vi "ReadGroupedDigitalOutputs.vi"(8 "error in (no error)":errorcluster, 11 "TesteractHAL_DigitalOutput_NIDAQmx In":refnum<class "TesteractHAL_DigitalOutput_NIDAQmx.lvclass">) -> (0 "error out":errorcluster, 2 "data":u32, 3 "TesteractHAL_DigitalOutput_NIDAQmx Out":refnum<class "TesteractHAL_DigitalOutput_NIDAQmx.lvclass">)   [LabVIEW 2017, in "TesteractHAL_DigitalOutput_NIDAQmx.lvlib" / "TesteractHAL_DigitalOutput_NIDAQmx.lvclass"]
doc: "Read a single channel."
uses:
  TesteractHAL_DigitalOutput_NIDAQmx.lvclass
  TesteractHAL_DigitalOutput_NIDAQmx.lvclass/TesteractHAL_DigitalOutput_NIDAQmx.ctl
  <vilib>/DAQmx/read.llb/DAQmx Read (Digital U32 1Chan 1Samp).vi
  <vilib>/DAQmx/miscellaneous.llb/DAQmx Fill In Error Info.vi
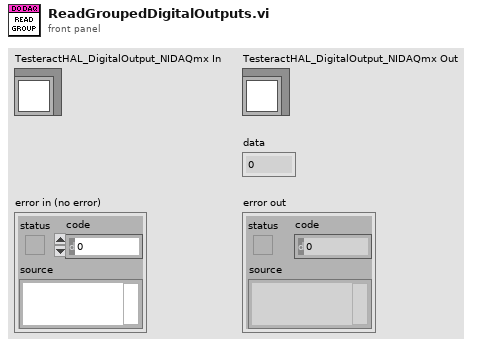
[diagram p1: front panel]
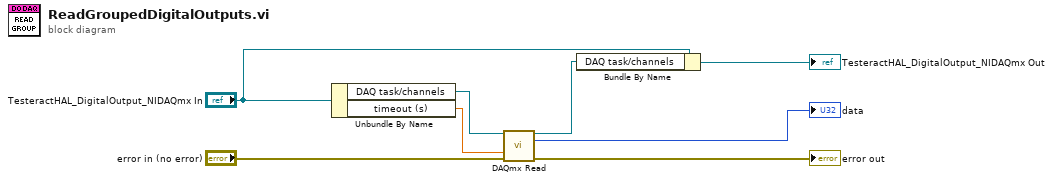
[diagram p0: block diagram]
diagram:
  n1 = Unbundle By Name("TesteractHAL_DigitalOutput_NIDAQmx In") -> ("DAQ task/channels"=w8:refnum<k21>, "timeout (s)"=w6:dbl)
  n2 = call-poly <vilib>:"DAQmx Read.vi"("task/channels in"=w8, "timeout"=w6, "error in"="error in (no error)") -> ("task out"=w7:refnum<k21>, "data"=→"data":u32, "error out"=→"error out":errorcluster)  [unwired: 10 in]
  n3 = Bundle By Name(cluster="TesteractHAL_DigitalOutput_NIDAQmx In", "DAQ task/channels"=w7) -> (→"TesteractHAL_DigitalOutput_NIDAQmx Out":refnum<class "TesteractHAL_DigitalOutput_NIDAQmx.lvclass">)
